vi "2_02.vi"() -> ()   [LabVIEW 2013]
uses:
  <vilib>/measure/NI_MABase.lvlib
  <vilib>/measure/NI_MAPro.lvlib
  <vilib>/measure/macond.llb/Continuous Waveform Convolution for 1 Chan.vi
  <vilib>/Analysis/NI_AALBase.lvlib
panel:
  out "Waveform Graph":dbl[](graph)
  in  "Frecuencia":dbl
  in  "Nivel de Ruido":dbl
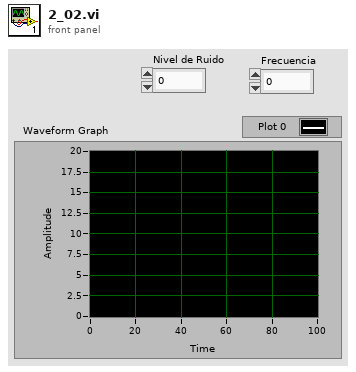
[diagram p1: front panel]
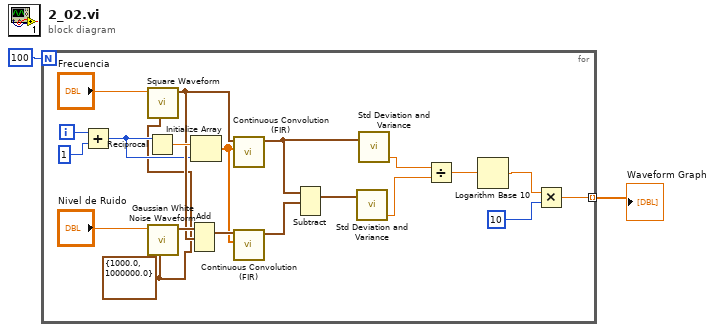
[diagram p0: block diagram]
diagram:
  n1 = for {
    N: 100 -> [_]
    tunnel: [w4] -> w1 mode=indexing
    i -> [w7]
    w3 = cluster{"Fs":dbl, "#s":dbl} {"Fs"=1000.0, "#s"=1000000.0} ("sampling info")
    n2 = Add(x=w7, y=1) -> (x+y=w5:i32)
    n3 = Reciprocal(x=w5) -> (1/x=w18:dbl)
    n4 = call <vilib>:"Square Waveform.vi"("sampling info"=w3, "frequency"="Frecuencia") -> ("signal out"=w16:waveform(dbl))  [unwired: 8 in, 1 out]
    n5 = call <vilib>:"Gaussian White Noise Waveform.vi"("sampling info"=w3, "standard deviation"="Nivel de Ruido") -> ("signal out"=w20:waveform(dbl))  [unwired: 8 in, 1 out]
    n6 = Add(1:w16, 2:w20) -> (0:w19:waveform(dbl))  [unwired: 1 in, 1 out]
    n7 = Initialize Array(w18, w5) -> (w17:dbl[])
    n8 = call-poly <vilib>:"Continuous Convolution (FIR).vi"("kernel"=w17, "signal in"=w16) -> ("signal out"=w13:waveform(dbl))  [unwired: 8 in, 1 out]
    n9 = call-poly <vilib>:"Continuous Convolution (FIR).vi"("kernel"=w17, "signal in"=w19) -> ("signal out"=w15:waveform(dbl))  [unwired: 8 in, 1 out]
    n10 = Subtract(1:w15, 2:w13) -> (0:w14:waveform(dbl))  [unwired: 1 in, 1 out]
    n11 = call <vilib>:"Std Deviation and Variance.vi"("X"=w14) -> ("variance"=w11:dbl)  [unwired: 1 in, 2 out]
    n12 = call <vilib>:"Std Deviation and Variance.vi"("X"=w13) -> ("variance"=w12:dbl)  [unwired: 1 in, 2 out]
    n13 = Divide(x=w12, y=w11) -> (x/y=w10:dbl)
    n14 = Logarithm Base 10(1:w10) -> (0:w9:dbl)
    n15 = Multiply(x=w9, y=10) -> (x*y=w4:dbl)
  }
  "Waveform Graph" <- w1
